vi "Rebuild Image for FPGA proc.vi"(11 "Array in":u8[](array[numeric])) -> (3 "Array out":u8[][](array[numeric]))   [LabVIEW 2015]
panel:
  out "output array":u8[][](graph)
  out "Numeric 2":i32
  out "Numeric":i32
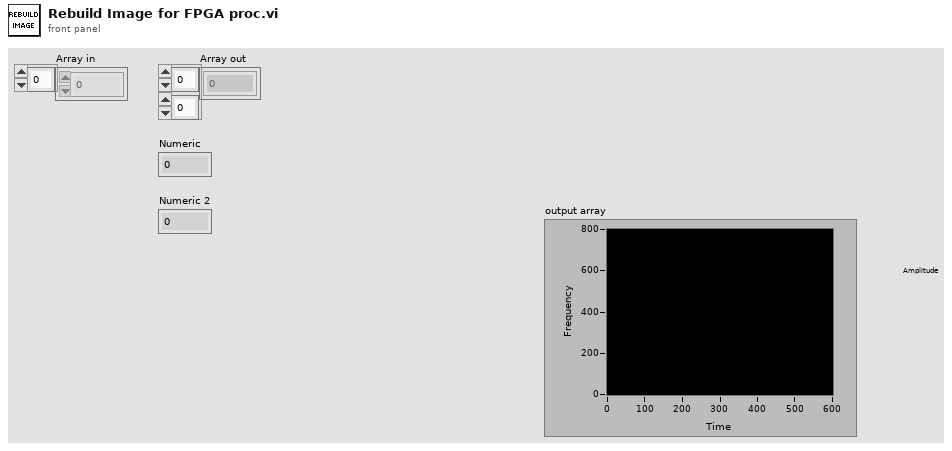
[diagram p1: front panel]
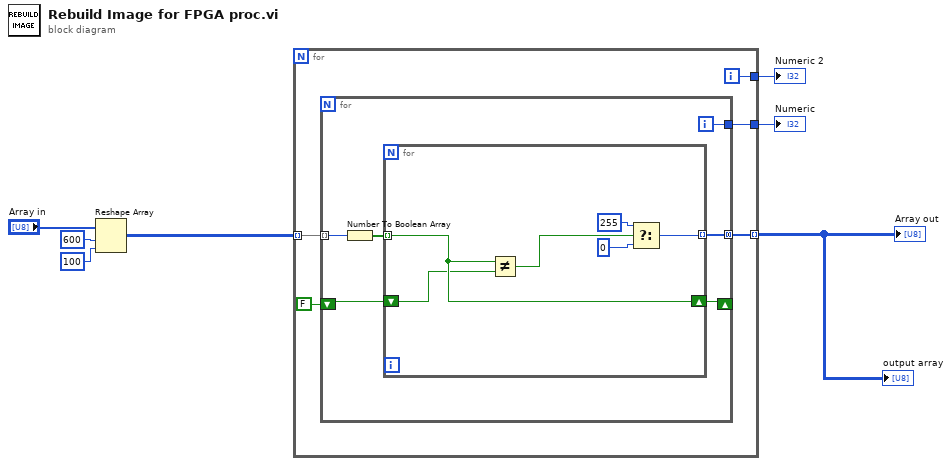
[diagram p0: block diagram]
diagram:
  n1 = Reshape Array("Array in", 600 ("dimension size"), 100 ("dimension size")) -> (w4:u8[][])
  n2 = for {
    tunnel: w4 -> [w12] mode=indexing
    tunnel: [w11] -> w1 mode=indexing
    tunnel: [w10] -> w3
    tunnel: [w9] -> w2
    i -> [w10]
    n3 = for {
      tunnel: w12 -> [w18] mode=indexing
      tunnel: [w16] -> w11 mode=concatenating
      tunnel: [w15] -> w9
      shift-right: [w14] -> _
      shift-left: FALSE -> [w13]
      i -> [w15]
      n4 = Number To Boolean Array(number=w18) -> (Boolean array=w17:bool[])
      n5 = for {
        tunnel: w17 -> [w21] mode=indexing
        tunnel: [w22] -> w16 mode=indexing
        shift-right: [w21] -> w14
        shift-left: w13 -> [w20]
        n6 = Not Equal?(x=w21, y=w20) -> (x != y?=w19:bool)
        n7 = Select(t=u8 255, s=w19, f=u8 0) -> (s? t:f=w22:u8)
      }
    }
  }
  "Numeric" <- w2
  "Numeric 2" <- w3
  "Array out" <- w1
  "output array" <- w1
